vi "TDMS Write.vi"(7 "Channel Name":string, 8 "error in (no error)":errorcluster, 9 "Group Name":string, 10 "TDMS in":refnum<k34>, 11 "Data Class in":refnum<class "Data Class.lvclass">) -> (0 "error out":errorcluster, 2 "TDMS Out":refnum<k34>)   [LabVIEW 2020, in "Data.lvlib" / "Data Class.lvclass"]
doc: "Write Generic Data to a TDMS file."
uses:
  Data Class.lvclass
  Data Class.lvclass/Data Class.ctl
  Cluster/Cluster.lvclass
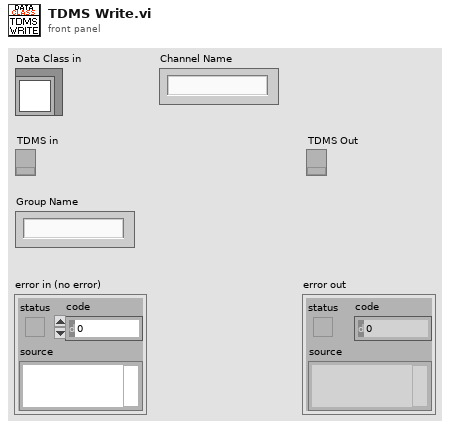
[diagram p1: front panel]
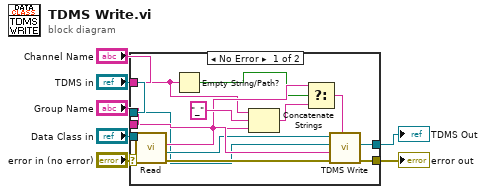
[diagram p0: block diagram]
diagram:
  n1 = case shown="No Error" "error in (no error)" {
    selector: "error in (no error)" -> [w20 w22]
    tunnel: [w13 w22] -> w1
    tunnel: "TDMS in" -> [w8 w23]
    tunnel: [w14 w23] -> w2
    tunnel: "Channel Name" -> [w12 _]
    tunnel: "Group Name" -> [w18 _]
    tunnel: "Data Class in" -> [w21 _]
    frame No Error {
      n2 = call "Read.vi"("error in (no error)"=w20, "Data Class in"=w21) -> ("error out"=w17:errorcluster, "Cluster"=w16:refnum<class "Cluster.lvclass">, "Class Alias"=w15:string)  [unwired: 6 in, 1 out]
      n3 = Empty String/Path?(string/path=w12) -> (empty?=w11:bool)
      n4 = Concatenate Strings(w12, "_" ("string"), w15) -> (w10:string)
      n5 = Select(t=w15, s=w11, f=w10) -> (s? t:f=w9:string)
      n6 = call-dynamic "TDMS Write.vi"("Channel Name"=w9, "error in (no error)"=w17, "Group Name"=w18, "TDMS in"=w8, "Cluster in"=w16) -> ("error out"=w13:errorcluster, "TDMS Out"=w14:refnum<k34>)  [unwired: 5 in]
    }
    frame Error {
    }
  }
  "error out" <- w1
  "TDMS Out" <- w2
